vi "Read number_of_tactics.vi"(8 "error in (no error)":errorcluster, 11 "PassBestReceiverRole in":refnum<class "PassBestReceiverRole.lvclass">) -> (0 "error out":errorcluster, 2 "number_of_tactics":dbl=2.0, 3 "PassBestReceiverRole out":refnum<class "PassBestReceiverRole.lvclass">)   [LabVIEW 2024, in "PassBestReceiverRole.lvclass"]
uses:
  PassBestReceiverRole.lvclass
  PassBestReceiverRole.lvclass/PassBestReceiverRole.ctl
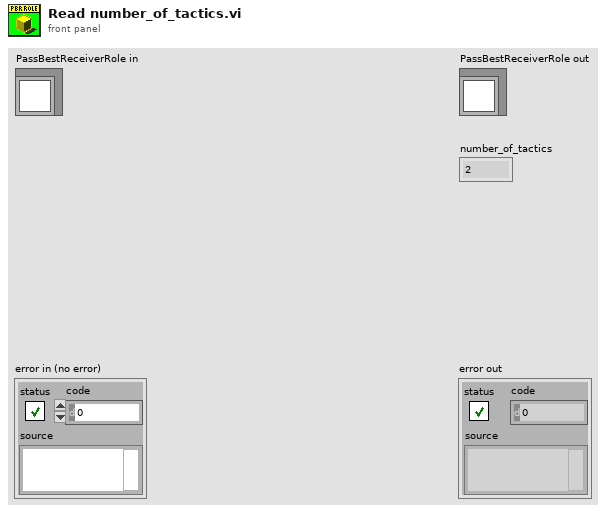
[diagram p1: front panel]
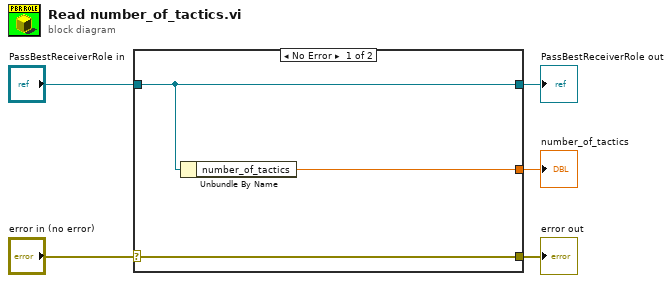
[diagram p0: block diagram]
diagram:
  n1 = case shown="No Error" "error in (no error)" {
    selector: "error in (no error)" -> [w8 w9]
    tunnel: [w8 w9] -> w4
    tunnel: [w7 w10] -> w2
    tunnel: "PassBestReceiverRole in" -> [w7 w10]
    tunnel: [w6 _] -> w1
    frame No Error {
      n2 = Unbundle By Name(w7) -> ("number_of_tactics"=w6:dbl)
    }
    frame Error {
    }
  }
  "error out" <- w4
  "PassBestReceiverRole out" <- w2
  "number_of_tactics" <- w1
